vi "Do.vi"(8 "error in (no error)":errorcluster, 10 "Actor in":refnum<class "Actor.lvclass">, 11 "Write tdms stream Msg":refnum<class "Write tdms stream Msg.lvclass">) -> (0 "error out":errorcluster, 2 "Actor out":refnum<class "Actor.lvclass">)   [LabVIEW 2021, in "Write tdms stream Msg.lvclass"]
doc: "This VI delivers the message to the actor by calling the appropriate method(s) on the actor."
uses:
  Write tdms stream Msg.lvclass
  <vilib>/ActorFramework/Actor/Actor.lvclass
  Template Module/Template Module.lvclass
  C:/Program Files/National Instruments/LabVIEW 2021/vi.lib/ActorFramework/Actor/Actor.lvclass
  Write tdms stream Msg.lvclass/Write tdms stream Msg.ctl
  Template Module/Template Module.lvclass/Template Module.ctl
  Template Module/Read tdms stream.vi
panel:
  out "NaN/Path/Refnum?":bool
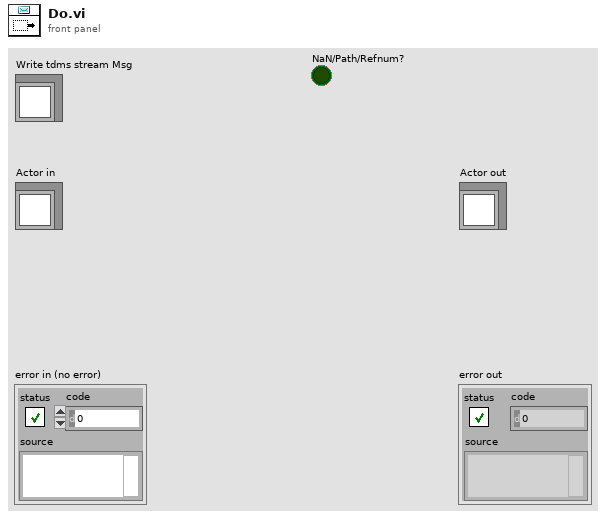
[diagram p1: front panel]
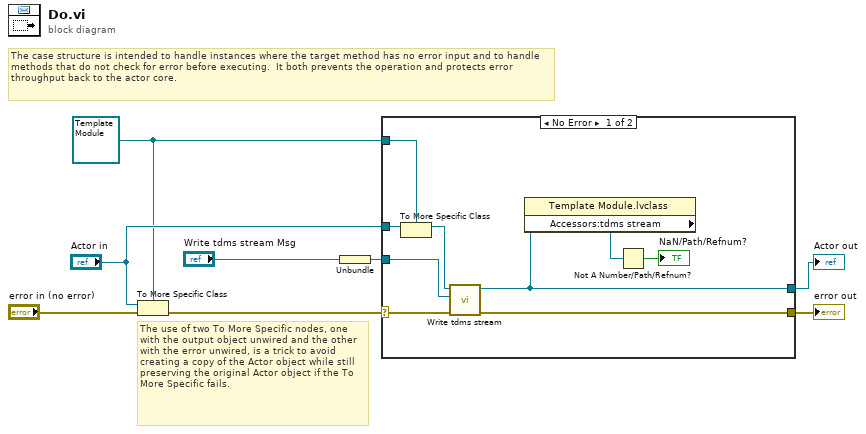
[diagram p0: block diagram]
diagram:
  w2 = refnum<class "Template Module.lvclass"> refnum ("Actor in")
  # "The use of two To More Specific nodes, one with the output object unwired and the other with the error unwired, is a trick to avoid creating a copy of the Actor object while still preserving the original Actor object if the To More Specific fails."
  # "The case structure is intended to handle instances where the target method has no error input and to handle methods that do not check for error before executing.  It both prevents the operation and protects error throughput back to the actor core."
  n1 = To More Specific Class(target class=w2, reference="Actor in", error in="error in (no error)") -> (error out=w6:errorcluster)  [unwired: 1 out]
  n2 = Unbundle("Write tdms stream Msg") -> (w1:refnum<k34>)
  n3 = case shown="No Error" w6 {
    selector: w6 -> [w16 w19]
    tunnel: [w17 w19] -> w5
    tunnel: [w12 w18] -> w4
    tunnel: "Actor in" -> [w15 w18]
    tunnel: w2 -> [w14 _]
    tunnel: w1 -> [w10 _]
    frame No Error {
      n4 = To More Specific Class(target class=w14, reference=w15) -> (specific class reference=w13:refnum<class "Template Module.lvclass">)  [unwired: 1 in, 1 out]
      n5 = call-dynamic "Write tdms stream.vi"("error in (no error)"=w16, "tdms stream"=w10, "Measure Object in"=w13) -> ("error out"=w17:errorcluster, "Measure Object out"=w12:refnum<class "Template Module.lvclass">)  [unwired: 7 in]
      n6 = property class="Template Module.lvclass"(reference=w12) -> ("Accessors:tdms stream"=w9:refnum<k34>)  [unwired: 1 in, 2 out]
      n7 = Not A Number/Path/Refnum?(number/path/refnum=w9) -> (NaN/Path/Refnum?=→"NaN/Path/Refnum?":bool)
    }
    frame Error {
      # "If type check fails, pass the original object out again."
    }
  }
  "error out" <- w5
  "Actor out" <- w4
